vi "MGCC_MdlMgmt_OpalRT_dynamic.vi"() -> ()   [LabVIEW 2016]
uses:
  <vilib>/imath/engines/lvmath2/RunTimeEngine/IndexRead/NIMS M($,S).vi
  <vilib>/imath/engines/lvmath2/RunTimeEngine/BuiltInFunctions/length/NIMS_length(GV).vi
  <vilib>/imath/engines/lvmath2/RunTimeEngine/BuiltInFunctions/zeros/NIMS_M=zeros(I32,I32).vi
  <vilib>/imath/engines/lvmath2/RunTimeEngine/ErrorHandling/NIMS_Create Error From Enums.vi
  <vilib>/imathl/engines/lvmath/Functions/Error Handling/Create Error.vi
  <vilib>/imath/engines/lvmath2/RunTimeEngine/IndexReplace/NIMS M(S,$)=V.vi
  <vilib>/imath/engines/lvmath2/RunTimeEngine/RangeToken/NIMS_Range_R3 - Integer.vi
  <vilib>/imath/engines/lvmath2/RunTimeEngine/IndexRead/NIMS M(S,S).vi
  <vilib>/imath/engines/lvmath2/RunTimeEngine/IndexRead/NIMS M(S,R2).vi
  <vilib>/imath/engines/lvmath2/RunTimeEngine/BuiltInFunctions/is_membermx/NIMS_is_membermx(GM,GM).vi
  <vilib>/imath/engines/lvmath2/RunTimeEngine/BuiltInFunctions/sum/NIMS_sum(GM,Sca).vi
  <vilib>/imath/engines/lvmath2/RunTimeEngine/IndexReplace/NIMS M(S,S)=S.vi
  <vilib>/imath/engines/lvmath2/RunTimeEngine/BuiltInFunctions/sum/NIMS_sum(GV).vi
  <vilib>/imath/engines/lvmath2/RunTimeEngine/BuiltInFunctions/findnz/NIMS_[1o]_findnz(GRowV).vi
  <vilib>/imath/engines/lvmath2/RunTimeEngine/IndexRead/NIMS M($,V).vi
  <vilib>/imath/engines/lvmath2/RunTimeEngine/BuiltInFunctions/sets_union/NIMS_sets_union(GV2).vi
  <vilib>/imath/engines/lvmath2/RunTimeSupport/NIMS_Get Any Vector_w Error - Matrix.vi
  <vilib>/imath/engines/lvmath2/RunTimeEngine/BuiltInFunctions/zeros/NIMS_V=zeros(I32,I32).vi
  <vilib>/imath/engines/lvmath2/RunTimeEngine/IndexReplace/NIMS M($,V)=V.vi
  <vilib>/imath/engines/lvmath2/RunTimeEngine/RangeToken/NIMS_Range.vi
  <vilib>/imath/engines/lvmath2/RunTimeEngine/CommandStatement/MC_CommandStatement_break.vi
  <vilib>/imath/engines/lvmath2/RunTimeEngine/BuiltInFunctions/is_membermx/NIMS_is_membermx(GV,GM).vi
  <vilib>/imath/engines/lvmath2/RunTimeEngine/BuiltInFunctions/findnz/NIMS_[1o]_findnz(GColV).vi
  <vilib>/imath/engines/lvmath2/RunTimeEngine/IndexRead/NIMS V(V).vi
  <vilib>/imath/engines/lvmath2/RunTimeEngine/IndexRead/NIMS M(M).vi
  <vilib>/imath/engines/lvmath2/RunTimeEngine/IndexReplace/NIMS M(S,S)=M.vi
  <vilib>/imath/engines/lvmath2/RunTimeSupport/NIMS_Error if Not Equal.vi
  <vilib>/imath/engines/lvmath2/RunTimeEngine/IndexReplace/NIMS V(S)=M.vi
  <vilib>/imath/engines/lvmath2/RunTimeEngine/IndexRead/NIMS V(S).vi
  <vilib>/imath/engines/lvmath2/RunTimeEngine/IndexReplace/NIMS V(S)=S.vi
  <vilib>/imath/engines/lvmath2/RunTimeEngine/IndexReplace/NIMS M(S,S)=V.vi
  <vilib>/imath/engines/lvmath2/RunTimeEngine/IndexReplace/NIMS V(S)=V.vi
  <vilib>/imath/engines/lvmath2/RunTimeEngine/IndexRead/NIMS M(R2,S).vi
  <vilib>/imath/engines/lvmath2/RunTimeSupport/NIMS_Get Scalar_w Error.vi
  <vilib>/imath/engines/lvmath2/RunTimeEngine/CommandStatement/NIMS_CommandStatement_MaskErr.vi
  <vilib>/imath/engines/lvmath2/RunTimeEngine/IndexRead/NIMS M(S,$).vi
  <vilib>/imath/engines/lvmath2/RunTimeEngine/IndexRead/NIMS V($).vi
  <vilib>/imath/engines/lvmath2/RunTimeEngine/IndexReplace/NIMS V(V)=V.vi
  <vilib>/imath/engines/lvmath2/RunTimeEngine/IndexReplace/NIMS M(V,V)=S.vi
  <vilib>/imath/engines/lvmath2/RunTimeEngine/IndexReplace/NIMS M(V,V)=V.vi
  <vilib>/imath/engines/lvmath2/RunTimeEngine/NodeEndStatement/NIMS_NodeEndStatement_Output.vi
  <vilib>/imath/engines/lvmath2/RunTimeEngine/ErrorHandling/NIMS_Finalize Error.vi
panel:
  out "Island_status":i32
  out "Energizematrix":dbl[](array[numeric])
  out "PQboundary":dbl[][](array[numeric])
  out "Array":dbl[][][](array[numeric])
  out "Line":dbl[][](array[numeric])
  out "Lineout":dbl[][](array[numeric])
  out "f_MGCC_MdlMgmt_Topology_RTDS":dbl[][](array[numeric])
  out "Node":dbl[][](array[numeric])
  out "error out":errorcluster
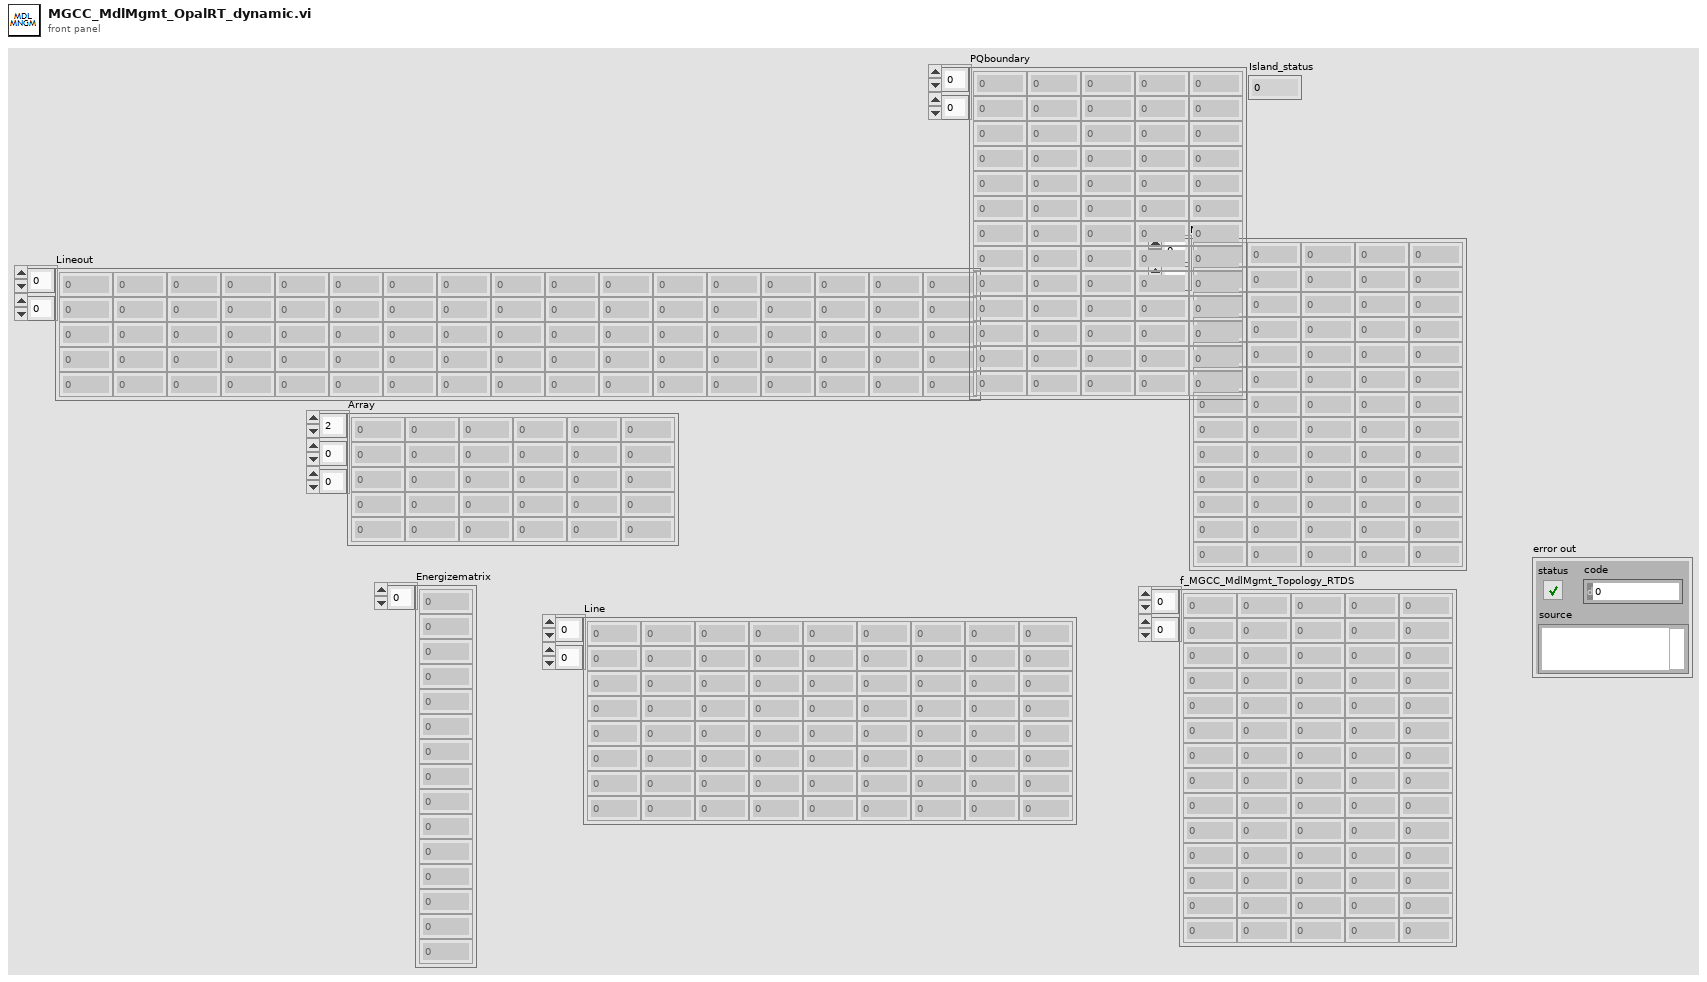
[diagram p1: front panel]
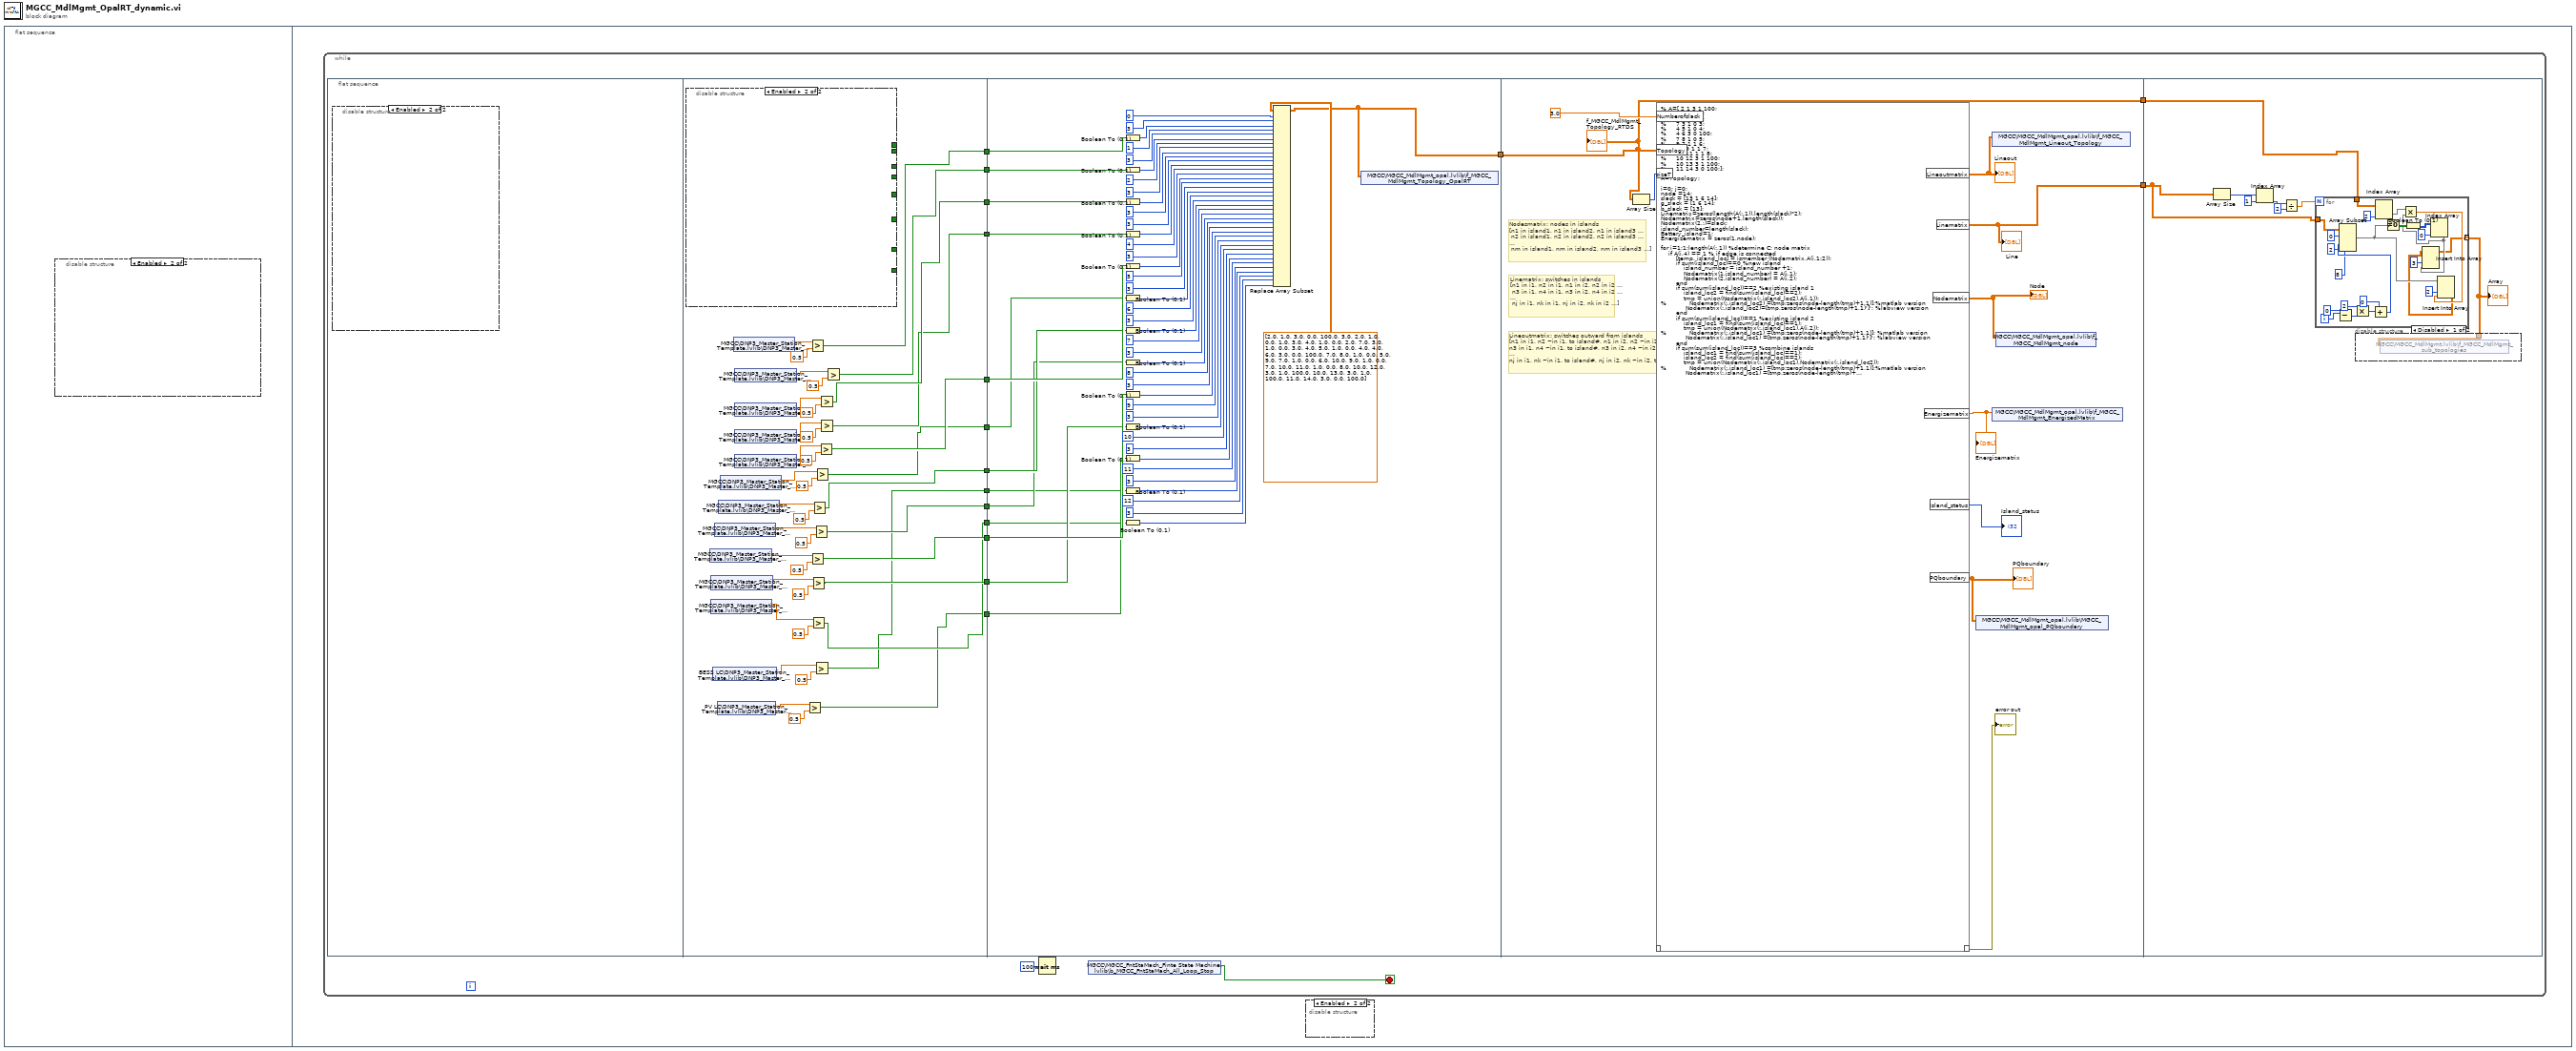
[diagram p0: block diagram]
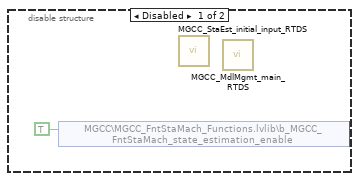
[diagram p2: hidden frame]
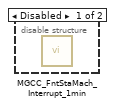
[diagram p3: hidden frame]
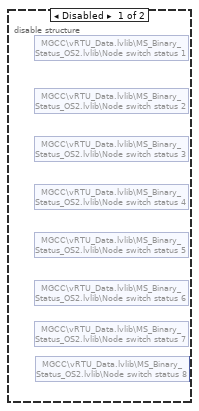
[diagram p4: hidden frame]
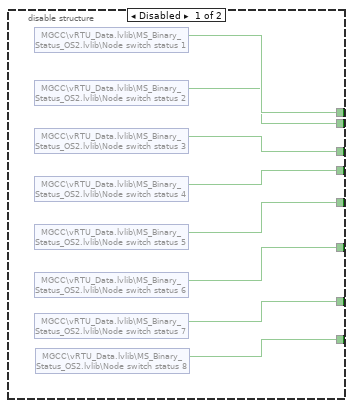
[diagram p5: hidden frame]
diagram:
  n1 = flat-sequence {
    frame #0 {
      n2 = disable-structure shown="Enabled" {
        frame Disabled {
          n3 = shared-variable "MGCC\\MGCC_FntStaMach_Functions.lvlib\\b_MGCC_FntStaMach_state_estimation_enable"(TRUE ("b_MGCC_FntStaMach_state_estimation_enable")) -> ()  [unwired: 1 in, 1 out]
          n4 = call "MGCC_StaEst_initial_input_RTDS.vi"() -> ()  [unwired: 12 in]
          n5 = call "MGCC_MdlMgmt_main_RTDS.vi"() -> ()  [unwired: 12 in]
        }
        frame Enabled {
        }
      }
    }
    frame #1 {
      n6 = while {
        stop <- w2 stop-if-true
        n7 = flat-sequence {
          tunnel: [w64] -> w17
          tunnel: [w52] -> w16
          tunnel: [w50] -> w15
          tunnel: [w48] -> w14
          tunnel: [w46] -> w13
          tunnel: [w44] -> w12
          tunnel: [w42] -> w11
          tunnel: [w40] -> w10
          tunnel: [w38] -> w9
          tunnel: [w36] -> w8
          tunnel: [w28] -> w7
          tunnel: [w29] -> w6
          tunnel: [w34] -> w5
          tunnel: w17 -> [w89]
          tunnel: w16 -> [w88]
          tunnel: w15 -> [w87]
          tunnel: w14 -> [w86]
          tunnel: w13 -> [w85]
          tunnel: w12 -> [w84]
          tunnel: w11 -> [w83]
          tunnel: w10 -> [w82]
          tunnel: w9 -> [w81]
          tunnel: w8 -> [w80]
          tunnel: w7 -> [w79]
          tunnel: w6 -> [w78]
          tunnel: w5 -> [w77]
          tunnel: [w75] -> w4
          tunnel: [w130] -> w18
          tunnel: w4 -> [w133]
          tunnel: [w133] -> w3
          tunnel: w18 -> [w3522]
          tunnel: w3 -> [w3521]
          frame #0 {
            n8 = disable-structure shown="Enabled" {
              frame Disabled {
                n9 = shared-variable "MGCC\\vRTU_Data.lvlib\\MS_Binary_Status_OS2.lvlib\\Node switch status 1"() -> (w27:bool)  [unwired: 1 in, 1 out]
                n10 = shared-variable "MGCC\\vRTU_Data.lvlib\\MS_Binary_Status_OS2.lvlib\\Node switch status 2"() -> (w26:bool)  [unwired: 1 in, 1 out]
                n11 = shared-variable "MGCC\\vRTU_Data.lvlib\\MS_Binary_Status_OS2.lvlib\\Node switch status 3"() -> (w25:bool)  [unwired: 1 in, 1 out]
                n12 = shared-variable "MGCC\\vRTU_Data.lvlib\\MS_Binary_Status_OS2.lvlib\\Node switch status 4"() -> (w24:bool)  [unwired: 1 in, 1 out]
                n13 = shared-variable "MGCC\\vRTU_Data.lvlib\\MS_Binary_Status_OS2.lvlib\\Node switch status 5"() -> (w23:bool)  [unwired: 1 in, 1 out]
                n14 = shared-variable "MGCC\\vRTU_Data.lvlib\\MS_Binary_Status_OS2.lvlib\\Node switch status 6"() -> (w22:bool)  [unwired: 1 in, 1 out]
                n15 = shared-variable "MGCC\\vRTU_Data.lvlib\\MS_Binary_Status_OS2.lvlib\\Node switch status 7"() -> (w21:bool)  [unwired: 1 in, 1 out]
                n16 = shared-variable "MGCC\\vRTU_Data.lvlib\\MS_Binary_Status_OS2.lvlib\\Node switch status 8"() -> (w20:bool)  [unwired: 1 in, 1 out]
              }
              frame Enabled {
              }
            }
          }
          frame #1 {
            n17 = disable-structure shown="Enabled" {
              disable-tunnel: [w74 _] -> _
              disable-tunnel: [w73 _] -> _
              disable-tunnel: [w72 _] -> _
              disable-tunnel: [w71 _] -> _
              disable-tunnel: [w70 _] -> _
              disable-tunnel: [w69 _] -> _
              disable-tunnel: [w68 _] -> _
              disable-tunnel: [w67 _] -> _
              frame Disabled {
                n18 = shared-variable "MGCC\\vRTU_Data.lvlib\\MS_Binary_Status_OS2.lvlib\\Node switch status 1"() -> (w70:bool)  [unwired: 1 in, 1 out]
                n19 = shared-variable "MGCC\\vRTU_Data.lvlib\\MS_Binary_Status_OS2.lvlib\\Node switch status 2"() -> (w69:bool)  [unwired: 1 in, 1 out]
                n20 = shared-variable "MGCC\\vRTU_Data.lvlib\\MS_Binary_Status_OS2.lvlib\\Node switch status 3"() -> (w68:bool)  [unwired: 1 in, 1 out]
                n21 = shared-variable "MGCC\\vRTU_Data.lvlib\\MS_Binary_Status_OS2.lvlib\\Node switch status 4"() -> (w67:bool)  [unwired: 1 in, 1 out]
                n22 = shared-variable "MGCC\\vRTU_Data.lvlib\\MS_Binary_Status_OS2.lvlib\\Node switch status 5"() -> (w74:bool)  [unwired: 1 in, 1 out]
                n23 = shared-variable "MGCC\\vRTU_Data.lvlib\\MS_Binary_Status_OS2.lvlib\\Node switch status 6"() -> (w73:bool)  [unwired: 1 in, 1 out]
                n24 = shared-variable "MGCC\\vRTU_Data.lvlib\\MS_Binary_Status_OS2.lvlib\\Node switch status 7"() -> (w72:bool)  [unwired: 1 in, 1 out]
                n25 = shared-variable "MGCC\\vRTU_Data.lvlib\\MS_Binary_Status_OS2.lvlib\\Node switch status 8"() -> (w71:bool)  [unwired: 1 in, 1 out]
              }
              frame Enabled {
              }
            }
            n26 = shared-variable "MGCC\\DNP3_Master_Station_Template.lvlib\\DNP3_Master_Data_Variables.lvlib\\MS_Analog_Status.lvlib\\S0910-status"() -> (w39:dbl)  [unwired: 1 in, 1 out]
            n27 = shared-variable "MGCC\\DNP3_Master_Station_Template.lvlib\\DNP3_Master_Data_Variables.lvlib\\MS_Analog_Status.lvlib\\S1114-status"() -> (w35:dbl)  [unwired: 1 in, 1 out]
            n28 = shared-variable "MGCC\\DNP3_Master_Station_Template.lvlib\\DNP3_Master_Data_Variables.lvlib\\MS_Analog_Status.lvlib\\S1011-status"() -> (w37:dbl)  [unwired: 1 in, 1 out]
            n29 = shared-variable "BESS LC\\DNP3_Master_Station_Template.lvlib\\DNP3_Master_Data_Variables.lvlib\\MS_Analog_Status.lvlib\\BESS-STATUS"() -> (w31:dbl)  [unwired: 1 in, 1 out]
            n30 = shared-variable "MGCC\\DNP3_Master_Station_Template.lvlib\\DNP3_Master_Data_Variables.lvlib\\MS_Analog_Status.lvlib\\S0709-status"() -> (w41:dbl)  [unwired: 1 in, 1 out]
            n31 = shared-variable "PV LC\\DNP3_Master_Station_Template.lvlib\\DNP3_Master_Data_Variables.lvlib\\MS_Analog_Status.lvlib\\PV-STATUS"() -> (w30:dbl)  [unwired: 1 in, 1 out]
            n32 = shared-variable "MGCC\\DNP3_Master_Station_Template.lvlib\\DNP3_Master_Data_Variables.lvlib\\MS_Analog_Status.lvlib\\S0708-status"() -> (w43:dbl)  [unwired: 1 in, 1 out]
            n33 = shared-variable "MGCC\\DNP3_Master_Station_Template.lvlib\\DNP3_Master_Data_Variables.lvlib\\MS_Analog_Status.lvlib\\S0406-status"() -> (w45:dbl)  [unwired: 1 in, 1 out]
            n34 = shared-variable "MGCC\\DNP3_Master_Station_Template.lvlib\\DNP3_Master_Data_Variables.lvlib\\MS_Analog_Status.lvlib\\S0102-status"() -> (w66:dbl)  [unwired: 1 in, 1 out]
            n35 = shared-variable "MGCC\\DNP3_Master_Station_Template.lvlib\\DNP3_Master_Data_Variables.lvlib\\MS_Analog_Status.lvlib\\S0203-status"() -> (w53:dbl)  [unwired: 1 in, 1 out]
            n36 = shared-variable "MGCC\\DNP3_Master_Station_Template.lvlib\\DNP3_Master_Data_Variables.lvlib\\MS_Analog_Status.lvlib\\S0304-status"() -> (w51:dbl)  [unwired: 1 in, 1 out]
            n37 = shared-variable "MGCC\\DNP3_Master_Station_Template.lvlib\\DNP3_Master_Data_Variables.lvlib\\MS_Analog_Status.lvlib\\S0307-status"() -> (w49:dbl)  [unwired: 1 in, 1 out]
            n38 = shared-variable "MGCC\\DNP3_Master_Station_Template.lvlib\\DNP3_Master_Data_Variables.lvlib\\MS_Analog_Status.lvlib\\S0405-status"() -> (w47:dbl)  [unwired: 1 in, 1 out]
            n39 = Greater?(x=w30, y=0.5) -> (0:w28:bool)
            n40 = Greater?(x=w66, y=0.5) -> (0:w64:bool)
            n41 = Greater?(x=w39, y=0.5) -> (0:w38:bool)
            n42 = Greater?(x=w37, y=0.5) -> (0:w36:bool)
            n43 = Greater?(x=w35, y=0.5) -> (0:w34:bool)
            n44 = Greater?(x=w43, y=0.5) -> (0:w42:bool)
            n45 = Greater?(x=w41, y=0.5) -> (0:w40:bool)
            n46 = Greater?(x=w31, y=0.5) -> (0:w29:bool)
            n47 = Greater?(x=w45, y=0.5) -> (0:w44:bool)
            n48 = Greater?(x=w47, y=0.5) -> (0:w46:bool)
            n49 = Greater?(x=w51, y=0.5) -> (0:w50:bool)
            n50 = Greater?(x=w49, y=0.5) -> (0:w48:bool)
            n51 = Greater?(x=w53, y=0.5) -> (0:w52:bool)
          }
          frame #2 {
            n52 = Boolean To (0,1)(Boolean=w89) -> (0, 1=w112:i16)
            n53 = Boolean To (0,1)(Boolean=w88) -> (0, 1=w111:i16)
            n54 = Boolean To (0,1)(Boolean=w87) -> (0, 1=w110:i16)
            n55 = Boolean To (0,1)(Boolean=w86) -> (0, 1=w109:i16)
            n56 = Boolean To (0,1)(Boolean=w85) -> (0, 1=w108:i16)
            n57 = Boolean To (0,1)(Boolean=w84) -> (0, 1=w107:i16)
            n58 = Boolean To (0,1)(Boolean=w83) -> (0, 1=w106:i16)
            n59 = Boolean To (0,1)(Boolean=w82) -> (0, 1=w105:i16)
            n60 = Boolean To (0,1)(Boolean=w81) -> (0, 1=w94:i16)
            n61 = Boolean To (0,1)(Boolean=w80) -> (0, 1=w93:i16)
            n62 = Boolean To (0,1)(Boolean=w79) -> (0, 1=w92:i16)
            n63 = Boolean To (0,1)(Boolean=w78) -> (0, 1=w91:i16)
            n64 = Boolean To (0,1)(Boolean=w77) -> (0, 1=w90:i16)
            n65 = Replace Array Subset(array=dbl[][] [[2.0, 1.0, 3.0, 0.0, 100.0], [3.0, 2.0, 1.0, 0.0, 1.0], [3.0, 4.0, 1.0, 0.0, 2.0], [7.0, 3.0, 1.0, 0.0, 3.0], [4.0, 5.0, 1.0, 0.0, 4.0], [4.0, 6.0, 3.0, 0.0, 100.0], [7.0, 8.0, 1.0, 0.0, 5.0], [9.0, 7.0, 1.0, 0.0, 6.0], [10.0, 9.0, 1.0, 0.0, 7.0], [10.0, 11.0, 1.0, 0.0, 8.0], [10.0, 12.0, 3.0, 1.0, 100.0], [10.0, 13.0, 3.0, 1.0, 100.0], [11.0, 14.0, 3.0, 0.0, 100.0]] ("f_MGCC_MdlMgmt_Topology_OpalRT"), new element #1=w112, index (row) #1=0 ("disabled index (row)"), index (col) #1=3 ("disabled index (col)"), new element #2=w111, index (row) #2=1 ("index (row)"), index (col) #2=3 ("disabled index (col)"), new element #3=w110, index (row) #3=2 ("index (row)"), index (col) #3=3 ("disabled index (col)"), new element #4=w109, index (row) #4=3 ("index (row)"), index (col) #4=3 ("disabled index (col)"), new element #5=w108, index (row) #5=4 ("index (row)"), index (col) #5=3 ("disabled index (col)"), new element #6=w107, index (row) #6=5 ("index (row)"), index (col) #6=3 ("disabled index (col)"), new element #7=w106, index (row) #7=6 ("index (row)"), index (col) #7=3 ("disabled index (col)"), new element #8=w105, index (row) #8=7 ("index (row)"), index (col) #8=3 ("disabled index (col)"), new element #9=w94, index (row) #9=8 ("index (row)"), index (col) #9=3 ("disabled index (col)"), new element #10=w93, index (row) #10=9 ("index (row)"), index (col) #10=3 ("disabled index (col)"), new element #11=w92, index (row) #11=10 ("index (row)"), index (col) #11=3 ("disabled index (col)"), new element #12=w91, index (row) #12=11 ("index (row)"), index (col) #12=3 ("disabled index (col)"), new element #13=w90, index (row) #13=12 ("index (row)"), index (col) #13=3 ("disabled index (col)")) -> (w75:dbl[][])
            n66 = shared-variable "MGCC\\MGCC_MdlMgmt_opal.lvlib\\f_MGCC_MdlMgmt_Topology_OpalRT"(w75) -> ()  [unwired: 1 in, 1 out]
          }
          frame #3 {
            # "Lineoutmatrix: switches outward from islands\n[n1 in i1, n2 ~in i1, to island#, n1 in i2, n2 ~in i2, to island#, ...\nn3 in i1, n4 ~in i1, to island#, n3 in i2, n4 ~in i2, to island#, ...\n...\nnj in i1, nk ~in i1, to island#, nj in i2, nk ~in i2, to island#, ...]"
            # "Linematrix: switches in islands\n[n1 in i1, n2 in i1, n1 in i2, n2 in i2 ...\n n3 in i1, n4 in i1, n3 in i2, n4 in i2 ...\n...\n nj in i1, nk in i1, nj in i2, nk in i2 ...]"
            # "Nodesmatrix: nodes in islands\n[n1 in island1, n1 in island2, n1 in island3 ...\n n2 in island1, n2 in island2, n2 in island3 ...\n...\n nm in island1, nm in island2, nm in island3 ...]"
            n67 = Array Size(array=w133) -> (size(s)=w137:i32[])
            n68 = mathscript code="% A=[ 2 1 3 1 100;\n%     3 2 1 0 1;\n%     3 4 1 0 2;\n%     7 3 1 0 3;\n%     4 5 1 0 4;\n%     4 6 3 0 100;\n%     7 8 1 0 5;\n%     9 7 1 1 6;\n%     10 9 1 1 7;\n%     10 11 1 1 8;\n%     10 12 3 1 100;\n%     10 13 3 1 100;\n%     11 14 3 0 100;];\n%     \nA=Topology;\n\ni=0; j=0;\nnode =14;\nslack = [13 1 6 14];\ng_slack = [1 6 14];\nb_slack = [13];\nLinematrix=zeros(length(A(:,1)),length(slack)*2);\nNodematrix=zeros(node+1,length(slack));\nNodematrix(2,:)=slack;\nisland_number=length(slack);\nBattery_island=1;\nEnergizematrix = zeros(1,node);\n\nfor i=1:1:length(A(:,1)) %determine C: node matrix\n    if A(i,4) == 1 % if edge is connected\n        [temp, island_loc] = ismember (Nodematrix,A(i,1:2));\n        if sum(island_loc)==0 %new island\n            island_number = island_number +1;\n            Nodematrix(1,island_number) = A(i,1);\n            Nodematrix(2,island_number) = A(i,2);\n        end\n        if sum(sum(island_loc))==2 %existing island 1\n            island_loc2 = find(sum(island_loc)==2);\n            tmp = union(Nodematrix(:,island_loc2),A(i,1));\n%            Nodematrix(:,island_loc2) =[tmp;zeros(node-length(tmp)+1,1)];%matlab version\n             Nodematrix(:,island_loc2)=[tmp,zeros(node-length(tmp)+1,1)']'; %labview version\n        end\n        if sum(sum(island_loc))==1 %existing island 2\n            island_loc1 = find(sum(island_loc)==1);\n            tmp = union(Nodematrix(:,island_loc1),A(i,2));\n%            Nodematrix(:,island_loc1) =[tmp;zeros(node-length(tmp)+1,1)]; %matlab version\n             Nodematrix(:,island_loc1) =[tmp,zeros(node-length(tmp)+1,1)']'; %labview version\n        end\n        if sum(sum(island_loc))==3 %combine islands\n            island_loc1 = find(sum(island_loc)==1);\n            island_loc2 = find(sum(island_loc)==2);\n            tmp = union(Nodematrix(:,island_loc1),Nodematrix(:,island_loc2));\n%            Nodematrix(:,island_loc1) =[tmp;zeros(node-length(tmp)+1,1)];%matlab version\n             Nodematrix(:,island_loc1) =[tmp,zeros(node-length(tmp)+1,1)']';%labview version\n            Nodematrix = Nodematrix(:,[1:island_loc2-1,island_loc2+1:end]);\n            island_number = island_number-1;\n        end\n    end\nend\n\n\nfor i=1:1:island_number %identify slack bus in nodes, and identify energized\n    [in_island, island_loc] = ismember(Nodematrix(:,i),b_slack);\n    if sum(in_island)~=0 %energized by battery\n        Nodematrix(1,i)=b_slack(island_loc(find(island_loc~=0,1,'first')));\n        Battery_island = i;\n        for j=1:1:node+1\n            if Nodematrix(j,i)~=0\n                Energizematrix(Nodematrix(j,i))=b_slack(island_loc(find(island_loc~=0,1,'first')));\n            end\n        end\n    end\n    [in_island, island_loc] = ismember(Nodematrix(:,i),g_slack);\n    if sum(in_island)==1 %energized by grid\n        Nodematrix(1,i)=g_slack(sum(island_loc));\n        for j=1:1:node+1\n            if Nodematrix(j,i)~=0\n                Energizematrix(Nodematrix(j,i))=g_slack(sum(island_loc));\n            end\n        end\n    end\n    if sum(in_island)>1 %two grid sources\n        Nodematrix(1,i)=g_slack(island_loc(find(island_loc~=0,1,'first')));\n        error_code = 10+i;\n        for j=1:1:node+1\n            if Nodematrix(j,i)~=0\n                Energizematrix(Nodematrix(j,i))=g_slack(island_loc(find(island_loc~=0,1,'first')));\n            end\n        end\n    end\n    if sum(in_island)==0 %no grid source\n\n    end\nend\n\nPQboundary = [0 0 0 0 0;0 0 0 0 0];\nPQboundary_index = 0;\nIsland_status = 0;\ntmp=Nodematrix(2:length(Nodematrix(:,1)),Battery_island);\ni=1;\nwhile i<=length(A(:,1)) %find out maximum boundary of battery island\n\n%     if A(i,4) == 0 % if edge not connected\n        [temp1, island_loc1] = ismember (tmp,A(i,1));\n        [temp2, island_loc2] = ismember (tmp,A(i,2));\n        if (sum(temp1)==1)&&(sum(temp2)==0)&&(Energizematrix(A(i,2))==0)\n            tmp = union(tmp,A(i,2));\n            i=1;\n        end\n        [temp, island_loc] = ismember (tmp,A(i,2));\n        if (sum(temp1)==0)&&(sum(temp2)==1)&&(Energizematrix(A(i,1))==0)\n            tmp = union(tmp,A(i,1));\n            i=1;\n        end\n%     end\n    i=i+1;\nend\nfor i=1:1:length(A(:,1))\n    [temp1, island_loc1] = ismember (tmp,A(i,1));\n    [temp2, island_loc2] = ismember (tmp,A(i,2));    \n    if (sum(temp1)~=0)&&(sum(temp2)~=0)\n        PQboundary_index = PQboundary_index +1;\n        PQboundary(PQboundary_index,:) = A(i,:);\n    \n    end\n   \nend\nfor i=1:1:length(g_slack(:))\n    [temp1, island_loc1] = ismember (tmp,g_slack(i));\n    if (sum(temp1)~=0)\n        Island_status=1;\n    end\nend\n        \n   \n\n\n\nLinematrix_index = zeros(1,island_number);\nLinematrix = zeros(1,island_number*2);\nLineoutmatrix_index = zeros(1,island_number);\nLineoutmatrix = zeros(1,island_number*4);\n\n\nfor i=1:1:length(A(:,1))\n    if A(i,4) == 1 % if edge is connected\n        [in_island, island_loc] = ismember (Nodematrix,A(i,1));\n        island_loc1 = find(sum(island_loc)~=0,1,'first');\n        Linematrix_index(island_loc1) = Linematrix_index(island_loc1)+1;\n        \n        Linematrix(Linematrix_index(island_loc1),island_loc1*2-1) = A(i,1);\n        Linematrix(Linematrix_index(island_loc1),island_loc1*2) = A(i,2);\n        \n%         if (Nodematrix(1,island_loc1) == b_slack(1))||(Energizematrix(A(i,1))==0)\n%             PQboundary_index = PQboundary_index +1;\n%             PQboundary(PQboundary_index,:) = A(i,:);\n%         end\n        \n        \n    end\n    if A(i,4) ==0 %if edge is not connected\n        island_loc1 = 0; island_loc2 = 0;\n        [in_island, island_loc] = ismember (Nodematrix,A(i,1));\n        island_loc1 = find(sum(island_loc)~=0,1,'first');\n        [in_island, island_loc] = ismember (Nodematrix,A(i,2));\n        island_loc2 = find(sum(island_loc)~=0,1,'first');\n        if island_loc1>0 %left terminal in island\n            Lineoutmatrix_index(island_loc1) = Lineoutmatrix_index(island_loc1) +1;\n            Lineoutmatrix(Lineoutmatrix_index(island_loc1),island_loc1*4-3) = i;\n            Lineoutmatrix(Lineoutmatrix_index(island_loc1),island_loc1*4-2) = A(i,1);\n            Lineoutmatrix(Lineoutmatrix_index(island_loc1),island_loc1*4-1) = A(i,2);\n            if island_loc2 > 0 %right terminal in island, critical line\n                Lineoutmatrix(Lineoutmatrix_index(island_loc1),island_loc1*4) = island_loc2;\n                \n                Lineoutmatrix_index(island_loc2) = Lineoutmatrix_index(island_loc2) +1;\n                Lineoutmatrix(Lineoutmatrix_index(island_loc2),island_loc2*4-3) = i;\n                Lineoutmatrix(Lineoutmatrix_index(island_loc2),island_loc2*4-2) = A(i,2);\n                Lineoutmatrix(Lineoutmatrix_index(island_loc2),island_loc2*4-1) = A(i,1);\n                Lineoutmatrix(Lineoutmatrix_index(island_loc2),island_loc2*4) = island_loc1;\n                \n            else %right terminal not in island, non critical line\n                Lineoutmatrix(Lineoutmatrix_index(island_loc2),island_loc2*4) = 0;\n                \n%                 if (Nodematrix(1,island_loc1) == b_slack(1))||(Energizematrix(A(i,1))==0)\n%                     PQboundary_index = PQboundary_index +1;\n%                     PQboundary(PQboundary_index,:) = A(i,:);\n%                 end\n            end\n        else %left terminal not in island\n            if island_loc2>0 %right terminal in island, non-critical line\n                Lineoutmatrix_index(island_loc2) = Lineoutmatrix_index(island_loc2) +1;\n                Lineoutmatrix(Lineoutmatrix_index(island_loc2),island_loc2*4-3) = i;\n                Lineoutmatrix(Lineoutmatrix_index(island_loc2),island_loc2*4-2) = A(i,2);\n                Lineoutmatrix(Lineoutmatrix_index(island_loc2),island_loc2*4-1) = A(i,1);\n                Lineoutmatrix(Lineoutmatrix_index(island_loc2),island_loc2*4) = 0;\n                \n%                 if (Nodematrix(1,island_loc2) == b_slack(1))||(Energizematrix(A(i,2))==0)\n%                     PQboundary_index = PQboundary_index +1;\n%                     PQboundary(PQboundary_index,:) = A(i,:);\n%                 end\n                \n            else %not in island, non-critical \n%                  [temp, island_loc] = ismember (tmp,A(i,1:2));\n%                  if sum(temp)~=0\n%                     PQboundary_index = PQboundary_index +1;\n%                     PQboundary(PQboundary_index,:) = A(i,:);\n%                  end\n            end\n        end\n    end\nend"("Numberofslack"=3.0, "Topology"=w133, "sizeT"=w137) -> ("??"=→"error out":errorcluster, "Linematrix"=w130:dbl[][], "Nodematrix"=w135:dbl[][], "PQboundary"=w134:dbl[][], "Energizematrix"=w132:dbl[], "Lineoutmatrix"=w131:dbl[][], "Island_status"=→"Island_status":i32)  [unwired: 1 in]
            "Node" <- w135
            "Lineout" <- w131
            "Line" <- w130
            "PQboundary" <- w134
            "Energizematrix" <- w132
            n69 = shared-variable "MGCC\\MGCC_MdlMgmt_opal.lvlib\\MGCC_MdlMgmt_opal_PQboundary"(w134) -> ()  [unwired: 1 in, 1 out]
            n70 = shared-variable "MGCC\\MGCC_MdlMgmt_opal.lvlib\\f_MGCC_MdlMgmt_EnergizedMatrix"(w132) -> ()  [unwired: 1 in, 1 out]
            n71 = shared-variable "MGCC\\MGCC_MdlMgmt_opal.lvlib\\f_MGCC_MdlMgmt_Lineout_Topology"(w131) -> ()  [unwired: 1 in, 1 out]
            n72 = shared-variable "MGCC\\MGCC_MdlMgmt_opal.lvlib\\f_MGCC_MdlMgmt_node"(w135) -> ()  [unwired: 1 in, 1 out]
            "f_MGCC_MdlMgmt_Topology_RTDS" <- w133
          }
          frame #4 {
            n73 = Array Size(array=w3522) -> (size(s)=w3528:i32[])
            n74 = Index Array(array=w3528, index=1) -> (element=w3526:i32)
            n75 = Divide(x=w3526, y=2) -> (x/y=w3524:dbl)
            n76 = for {
              N: w3524 -> [_]
              tunnel: w3522 -> [w3553]
              tunnel: [w3530] -> w3523 mode=indexing
              tunnel: w3521 -> [w3538]
              i -> [w3551]
              n77 = Subtract(x=w3551, y=0) -> (x-y=w3549:i32)
              n78 = Multiply(x=2, y=w3549) -> (x*y=w3547:i32)
              n79 = Add(x=w3547, y=0) -> (x+y=w3545:i32)
              n80 = Array Subset(array=w3553, index (row)=0 ("index"), length (row)=8 ("length"), index (col)=w3545, length (col)=2 ("length")) -> (w3532:dbl[][])
              n81 = Index Array(array=w3538, index (col)=2 ("disabled index (col)")) -> (element=w3536:dbl[])  [unwired: 1 in]
              n82 = Not Equal To 0?(x=w3532) -> (x != 0?=w3542:bool[][])
              n83 = Boolean To (0,1)(Boolean=w3542) -> (0, 1=w3541:i16[][])
              n84 = Index Array(array=w3541, index (col)=0 ("disabled index (col)")) -> (element=w3535:i16[])  [unwired: 1 in]
              n85 = Multiply(x=w3536, y=w3535) -> (x*y=w3534:dbl[])
              n86 = Insert Into Array(array=w3532, index (col)=2 ("disabled index (col)"), new element=w3534) -> (w3531:dbl[][])  [unwired: 1 in]
              n87 = Insert Into Array(array=w3531, index (col)=3 ("disabled index (col)"), new element=w3535) -> (w3530:dbl[][])  [unwired: 1 in]
            }
            "Array" <- w3523
            n88 = disable-structure shown="Disabled" {
              disable-tunnel: w3523 -> [w3529 _]
              frame Disabled {
                n89 = shared-variable "MGCC\\MGCC_MdlMgmt.lvlib\\f_MGCC_MdlMgmt_sub_topologies"(w3529) -> ()  [unwired: 1 in, 1 out]
              }
              frame Enabled {
              }
            }
          }
        }
        n90 = Wait (ms)(milliseconds to wait=u32 100) -> ()  [unwired: 1 out]
        n91 = shared-variable "MGCC\\MGCC_FntStaMach_Finte State Machine.lvlib\\b_MGCC_FntStaMach_All_Loop_Stop"() -> (w2:bool)  [unwired: 1 in, 1 out]
      }
      n92 = disable-structure shown="Enabled" {
        frame Disabled {
          n93 = call "MGCC_FntStaMach_Interrupt_1min.vi"() -> ()  [unwired: 11 in, 1 out]
        }
        frame Enabled {
        }
      }
    }
  }
